vi "Count_looped_sub.vi"(7 "Reset?":bool, 11 "Input sample":dbl format="%#_13g") -> (3 "Sum of samples":dbl)   [LabVIEW 2018]
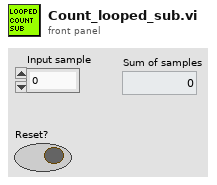
[diagram p1: front panel]
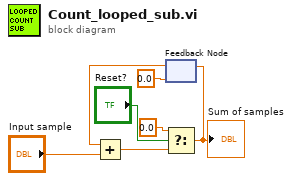
[diagram p0: block diagram]
diagram:
  n1 = feedback #1(0.0) -> (w2:dbl)
  n2 = Add(x=w2, y="Input sample") -> (x+y=w4:dbl)
  n3 = Select(t=0.0, s="Reset?", f=w4) -> (s? t:f=w3:dbl)
  "Sum of samples" <- w3
  n4 = feedback-in #1(w3) -> ()
